vi "setData.vi"(8 "error in (no error)":errorcluster, 10 "ContextData.lvclass":refnum<class "ContextData.lvclass">, 11 "Context in":refnum<class "Context.lvclass">) -> (0 "error out":errorcluster, 3 "Context out":refnum<class "Context.lvclass">)   [LabVIEW 2018, in "Context.lvclass"]
uses:
  Context.lvclass
  ContextData/ContextData.lvclass
  Context.lvclass/Context.ctl
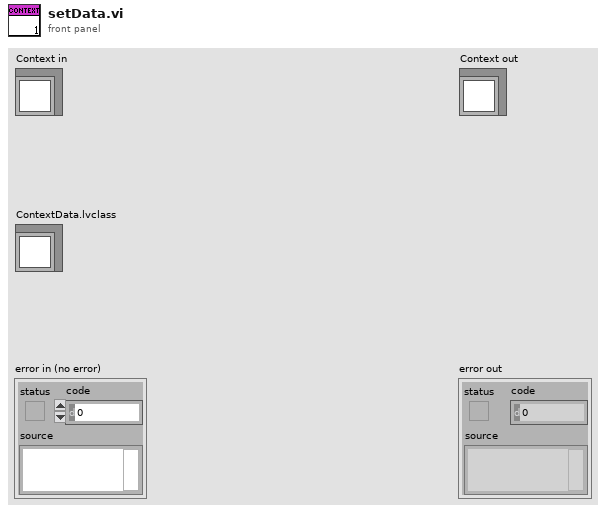
[diagram p1: front panel]
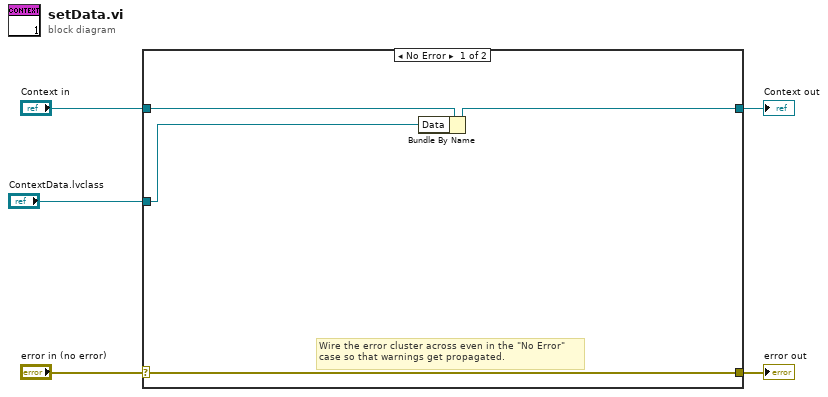
[diagram p0: block diagram]
diagram:
  n1 = case shown="No Error" "error in (no error)" {
    selector: "error in (no error)" -> [w8 w11]
    tunnel: [w8 w11] -> w4
    tunnel: [w7 w10] -> w2
    tunnel: "Context in" -> [w9 w10]
    tunnel: "ContextData.lvclass" -> [w6 _]
    frame No Error {
      # "Wire the error cluster across even in the \"No Error\"\ncase so that warnings get propagated."
      n2 = Bundle By Name(cluster=w9, "Data"=w6) -> (w7:refnum<class "Context.lvclass">)
    }
    frame Error {
    }
  }
  "error out" <- w4
  "Context out" <- w2
